vi "Set Configuration.vi"(7 "Detector Manager":refnum<class "Detector Manager.lvclass">, 8 "error in (no error)":errorcluster, 10 "Configuration Name":string, 11 "Father Of All Detectors in":refnum<class "Father Of All Detectors.lvclass">) -> (0 "error out":errorcluster, 3 "Father Of All Detectors out":refnum<class "Father Of All Detectors.lvclass">)   [LabVIEW 2026, in "TALOS.lvlib" / "Father Of All Detectors.lvlib" / "Father Of All Detectors.lvclass"]
uses:
  Father Of All Detectors.lvclass
  Internal uServices/System uServices/Detector Manager/Detector Manager/Detector Manager.lvclass
  C:/LabVIEW Code/TALOS/talos/Ancestor/Ancestor/Ancestor.lvclass
  C:/LabVIEW Code/TALOS/talos/Father of all uServices/Father of all uServices/Father of all uServices.lvclass
  Father Of All Detectors.lvclass/Father Of All Detectors.ctl
  Ancestor/Ancestor/Ancestor.lvclass/Ancestor.ctl
  Guardian/Guardian Messages/Message to uService Msg/Message to uService Msg.lvclass/Message to uService Msg.ctl
  Ancestor/Ancestor/Read ID.vi
  Father of all uServices/Father of all uServices/Children Methods/Message to uService.vi
  Support VIs/Generate Error.vi
  Guardian/Guardian Messages/Message to uService Msg/Send Message to uService.vi
  FGV/Error Memory/Get Error Description.vi
  Support VIs/Get PC name.vi
  Support VIs/Get Class Name.vi
  FGV/Error Memory/Error Memory Core.vi
  <vilib>/AdvancedString/Delimited String to 1D String Array.vi
  <vilib>/AdvancedString/Delimited String to 1D String Array (string).vi
  Support VIs/Circus Root Path.vi
  FGV/Error Memory/Error Crt Lvl checker.vi
  FGV/Error Memory/Error Memory Core.vi/40c8088d-b597-4017-91af-faa98e00292e.vi
  FGV/Error Memory/Error Memory Core.vi/d4a3ab98-063c-4e44-b43d-fbdcfe6c2be2.vi
  Father of all uServices/Father of all uServices/Father of all uServices.lvclass
  C:/LabVIEW Code/TALOS/builds/Actor Framework PPL/Actor Framework.lvlibp/1abvi3w/vi.lib/ActorFramework/Actor/Actor.lvclass
  Support VIs/Global Memory.vi
  builds/Actor Framework PPL/Actor Framework.lvlibp/1abvi3w/vi.lib/ActorFramework/Actor/Read Caller Enqueuer.vi
  builds/Actor Framework PPL/Actor Framework.lvlibp/1abvi3w/vi.lib/ActorFramework/Message Enqueuer/Enqueue.vi
  <vilib>/Utility/LVClass/Get LV Class Name.vi
  Support VIs/Is in Packed Library.vi
  Support VIs/TALOS Root path.vi
  Support VIs/Read CSV worksheet.vi
  Support VIs/Global Constants.vi
  <vilib>/Utility/error.llb/General Error Handler.vi
  Support VIs/Error Log.vi
  Guardian/Guardian Messages/Message to uService Msg/Message to uService Msg.lvclass
  Ancestor/Ancestor/Ancestor.lvclass
  <vilib>/Comparison/Equal/Equal Functor/Equal Functor.lvclass
  Config/Config.lvclass
  TALOS.lvlib
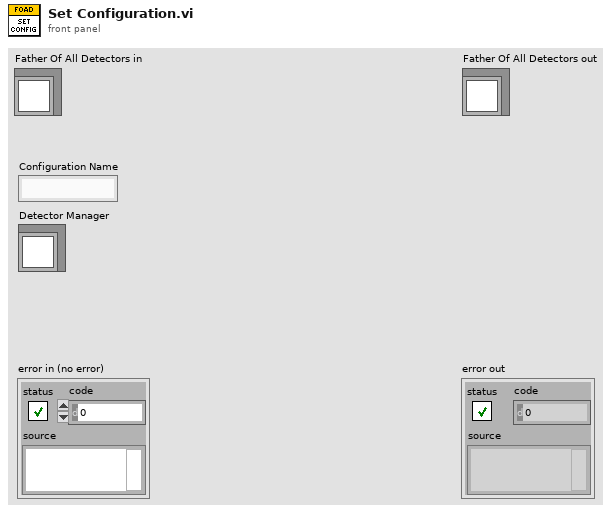
[diagram p1: front panel]
types:
  T1 = cluster{"Configuration Name ":string, "All parameters":string[][]}
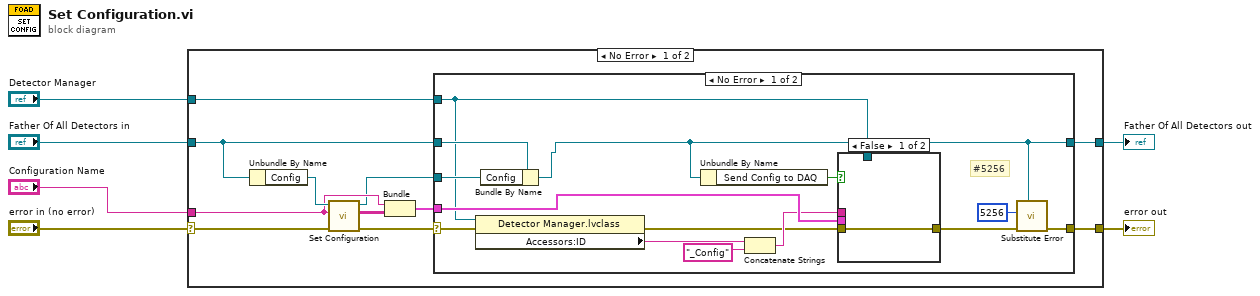
[diagram p0: block diagram]
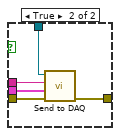
[diagram p2: hidden frame]
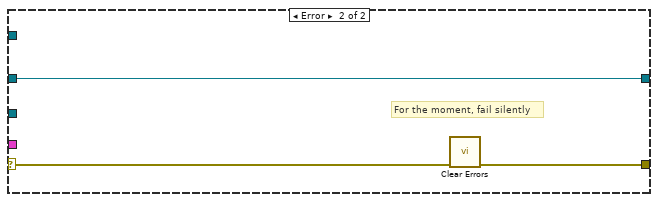
[diagram p3: hidden frame]
diagram:
  n1 = case shown="No Error" "error in (no error)" {
    selector: "error in (no error)" -> [w16 w42]
    tunnel: [w10 w42] -> w5
    tunnel: [w9 w41] -> w3
    tunnel: "Father Of All Detectors in" -> [w15 w41]
    tunnel: "Configuration Name" -> [w13 _]
    tunnel: "Detector Manager" -> [w7 _]
    frame No Error {
      n2 = Unbundle By Name(w15) -> ("Config"=w17:refnum<class "Config.lvclass">)
      n3 = call-dynamic "Set Configuration.vi"("error in (no error)"=w16, "Config name"=w13, "Config in"=w17) -> ("error out"=w14:errorcluster, "All parameters"=w12:string[][], "Config out"=w8:refnum<class "Config.lvclass">)  [unwired: 6 in]
      n4 = Bundle("Configuration Name"=w13, "All parameters"=w12) -> (w11:T1)  [unwired: 1 in]
      n5 = case shown="No Error" w14 {
        selector: w14 -> [w22 w40]
        tunnel: w15 -> [w21 w39]
        tunnel: w11 -> [w31 _]
        tunnel: [w29 w38] -> w10
        tunnel: [w23 w39] -> w9
        tunnel: w8 -> [w25 _]
        tunnel: w7 -> [w20 _]
        frame No Error {
          # "#5256"
          n6 = property class="Detector Manager.lvclass"(reference=w20, error in=w22) -> (error out=w18:errorcluster, "Accessors:ID"=w19:string)  [unwired: 1 out]
          n7 = Bundle By Name(cluster=w21, "Config"=w25) -> (w23:refnum<class "Father Of All Detectors.lvclass">)
          n8 = Unbundle By Name(w23) -> ("Send Config to DAQ"=w24:bool)
          n9 = Concatenate Strings(w19, "_Config" ("string")) -> (w27:string)
          n10 = case shown="False" w24 {
            tunnel: w31 -> [_ w36]
            tunnel: [w32 w37] -> w30
            tunnel: w27 -> [_ w35]
            tunnel: w20 -> [_ w34]
            tunnel: w18 -> [w32 w33]
            frame False {
            }
            frame True {
              n11 = call "Send to DAQ.vi"("error in (no error)"=w33, "Data"=w36, "Data Name"=w35, "Father of all uServices in"=w34) -> ("error out"=w37:errorcluster)  [unwired: 6 in, 1 out]
            }
          }
          n12 = call "Substitute Error.vi"("LabVIEW Object"=w23, "error in (no error)"=w30, "Error Code"=5256) -> ("error out"=w29:errorcluster)  [unwired: 8 in]
        }
        frame Error {
          # "For the moment, fail silently"
          n13 = call <vilib>:"Clear Errors.vi"("error in (no error)"=w40) -> ("error out"=w38:errorcluster)  [unwired: 5 in, 1 out]
        }
      }
    }
    frame Error {
    }
  }
  "error out" <- w5
  "Father Of All Detectors out" <- w3
